vi "Get index from key.vi"(8 "error in (no error)":errorcluster, 9 "value":string, 10 "key":string, 11 "VElement":variant) -> (0 "error out":errorcluster, 3 "indexOut":i32)   [LabVIEW 2015]
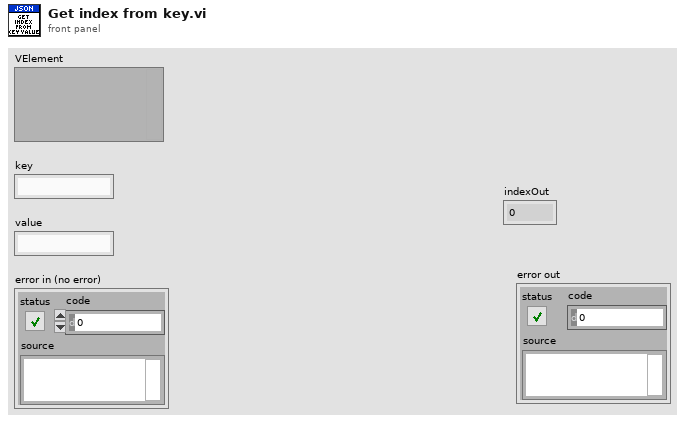
[diagram p1: front panel]
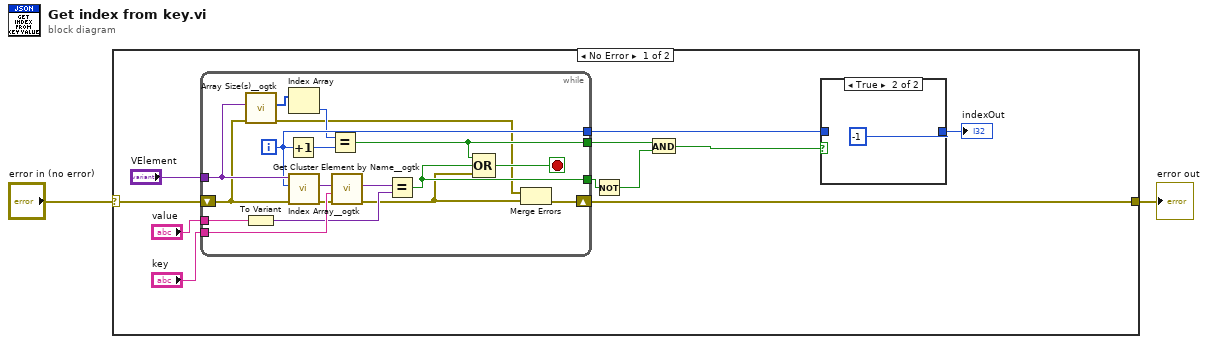
[diagram p0: block diagram]
diagram:
  n1 = case shown="No Error" "error in (no error)" {
    selector: "error in (no error)" -> [w12 w34]
    tunnel: [w9 w34] -> w1
    frame No Error {
      n2 = while {
        tunnel: "VElement" -> [w29]
        tunnel: "key" -> [w32]
        tunnel: "value" -> [w31]
        tunnel: [w27] -> w5
        shift-right: [w17] -> w9
        shift-left: w12 -> [w19]
        tunnel: [w22] -> w7
        tunnel: [w21] -> w8
        i -> [w27]
        stop <- w20 stop-if-true
        n3 = call <userlib>:"Array Size(s)__ogtk.vi"("error in (no error)"=w19, "Array"=w29) -> ("error out"=w16:errorcluster, "Size(s)"=w28:u32[])  [unwired: 7 in, 1 out]
        n4 = To Variant(anything=w31) -> (Variant=w23:variant)
        n5 = Increment(x=w27) -> (x+1=w25:i32)
        n6 = Index Array(array=w28) -> (element=w26:u32)  [unwired: 1 in]
        n7 = call <userlib>:"Index Array__ogtk.vi"("error in (no error)"=w19, "Index (1D)"=w27, "MultiD Array"=w29) -> ("error out"=w30:errorcluster, "Array Element"=w33:variant)  [unwired: 7 in]
        n8 = Equal?(x=w26, y=w25) -> (x = y?=w22:bool)
        n9 = call <userlib>:"Get Cluster Element by Name__ogtk.vi"("error in (no error)"=w30, "Element Name"=w32, "Cluster"=w33) -> ("error out"=w18:errorcluster, "VElement"=w24:variant)  [unwired: 6 in, 1 out]
        n10 = Equal?(x=w24, y=w23) -> (x = y?=w21:bool)
        n11 = Compound Arithmetic op=OR(w22, w21, w18) -> (w20:bool)
        n12 = Merge Errors(w16, w18) -> (w17:errorcluster)
      }
      n13 = Not(x=w8) -> (.not. x?=w6:bool)
      n14 = And(x=w7, y=w6) -> (x .and. y?=w3:bool)
      n15 = case shown="True" w3 {
        tunnel: [w14 -1] -> w4
        tunnel: w5 -> [w14 _]
        frame False {
        }
        frame True {
        }
      }
      "indexOut" <- w4
    }
    frame Error {
    }
  }
  "error out" <- w1
